vi "MHL_load file.vi"(0 "Data Cluster in":T1, 5 "error in (no error)":errorcluster) -> (14 "Data Cluster out":T1, 15 "Size (bytes)":i64=37399506 format="%.0p", 19 "error out":errorcluster)   [LabVIEW 2019, in "Main UI.lvlib"]
uses:
  Main UI.lvlib
  Module Data--cluster.ctl
  Neo-Laura-LVOOP/Class Library/XYgraph_class/XYgraph.lvclass
  FileReader/FPref_clustered--cluster references.ctl
  Main UI Shared/Boolean--FP cluster.ctl
  FileReader/FPref_cntrls--cluster references.ctl
  Main UI Shared/Indicators--FP cluster.ctl
  FileReader/FileReader.lvlib
  Analysis/Analysis.lvlib
  Main UI Shared/MAIN UI Shared.lvlib
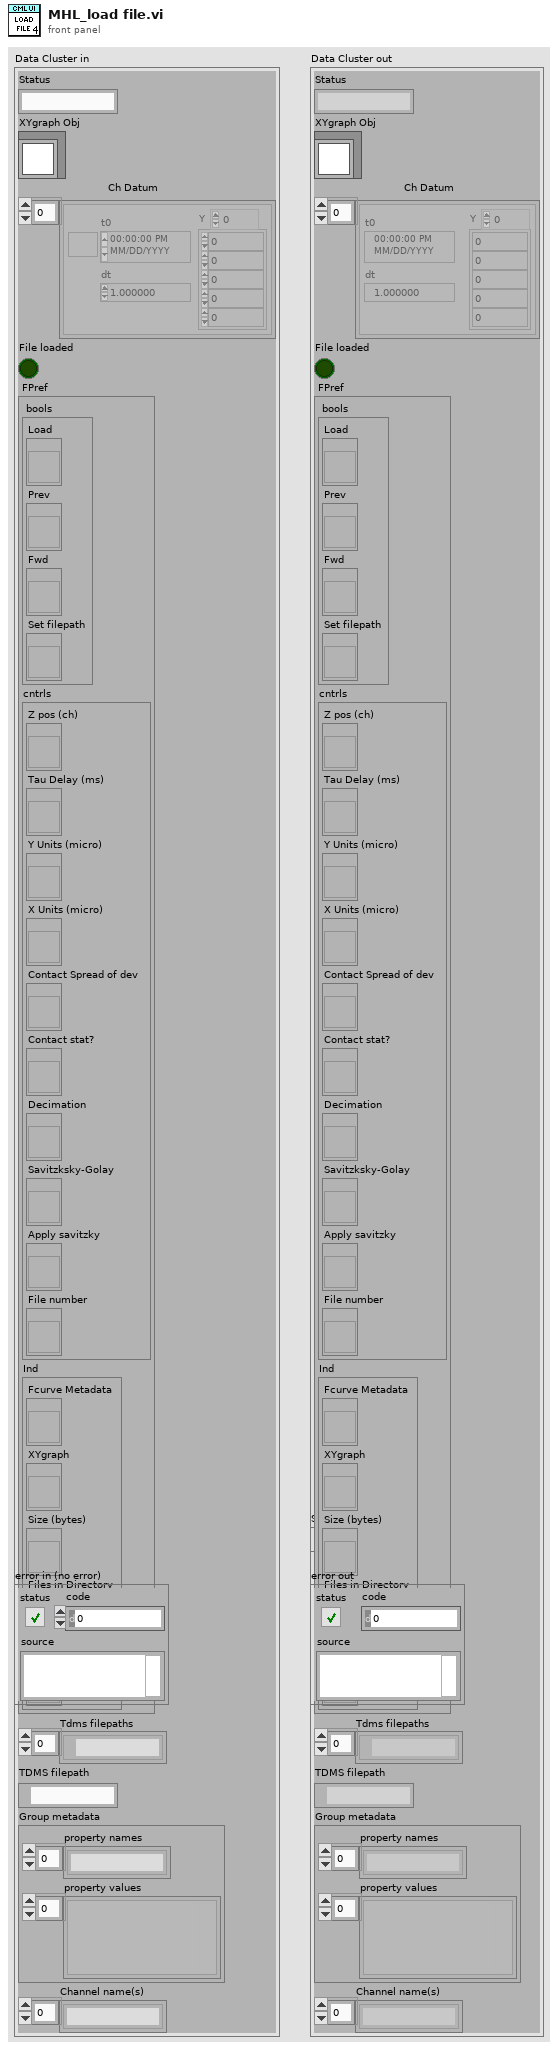
[diagram p1: front panel]
types:
  T1 = typedef "Main UI.lvlib/Module Data--cluster.ctl" = cluster{"Status":string, "XYgraph Obj":refnum<class "XYgraph.lvclass">, "Ch Datum":waveform(dbl)[], "File loaded":bool, "FPref":T2, "Tdms filepaths":path[], "TDMS filepath":path, "Group metadata":cluster{"property names":string[], "property values":variant[]}, "Channel name(s)":string[]}
  T2 = typedef "FPref_clustered--cluster references.ctl" = cluster{" bools":T3, "cntrls":T4, "Ind":T5}
  T3 = typedef "MAIN UI Shared.lvlib/Boolean--FP cluster.ctl" = cluster{"Load":refnum<vi>, "Prev":refnum<vi>, "Fwd":refnum<vi>, "Set filepath":refnum<vi>}
  T4 = typedef "FPref_cntrls--cluster references.ctl" = cluster{"Z pos (ch)":refnum<vi>, "Tau Delay (ms)":refnum<vi>, "Y Units (micro)":refnum<vi>, "X Units (micro)":refnum<vi>, "Contact Spread of dev":refnum<vi>, "Contact stat?":refnum<vi>, "Decimation":refnum<vi>, "Savitzksky-Golay":refnum<vi>, "Apply savitzky ":refnum<vi>, "File number":refnum<vi>}
  T5 = typedef "Indicators--FP cluster.ctl" = cluster{"Fcurve Metadata":refnum<vi>, "XYgraph":refnum<vi>, "Size (bytes)":refnum<vi>, "Files in Directory":refnum<vi>, "Filepath":refnum<vi>}
  T6 = typedef "MAIN UI Shared.lvlib/Apply_Savitsky--cluster.ctl" = cluster{"Def":bool, "Zpos":bool}
  T7 = typedef "FileReader.lvlib/Open TDMS file (Reply Payload)--cluster.ctl" = cluster{"Group metadata":T8, "Channel name(s)":string[], "Channel datum out":waveform(dbl)[], "size (in bytes)":i64, "error":errorcluster}
  T8 = typedef "TDMS_DataHandler.lvclass/Fcurve Meta data.ctl" = cluster{"property names":string[], "property values":variant[]}
  T9 = typedef "XYgraph.lvclass/Units --enum.ctl" = string
  T10 = typedef "Fcurve.lvclass/Metadata.ctl" = cluster{"dt (us)":dbl, "Dec Factor":dbl, "Z piezo Sensitivity (nm/V)":dbl, "K (N/m)":dbl, "Sp (V)":dbl, "Contact (ms)":dbl, "Zpos contact":dbl, "Vel_app (nm/s)":dbl, "Vel_ret (nm/s)":dbl, "deltaV (nm)":dbl, "Def_V0 (v)":dbl, "Piezo gain":dbl, "invOLS (nm/V)":dbl}
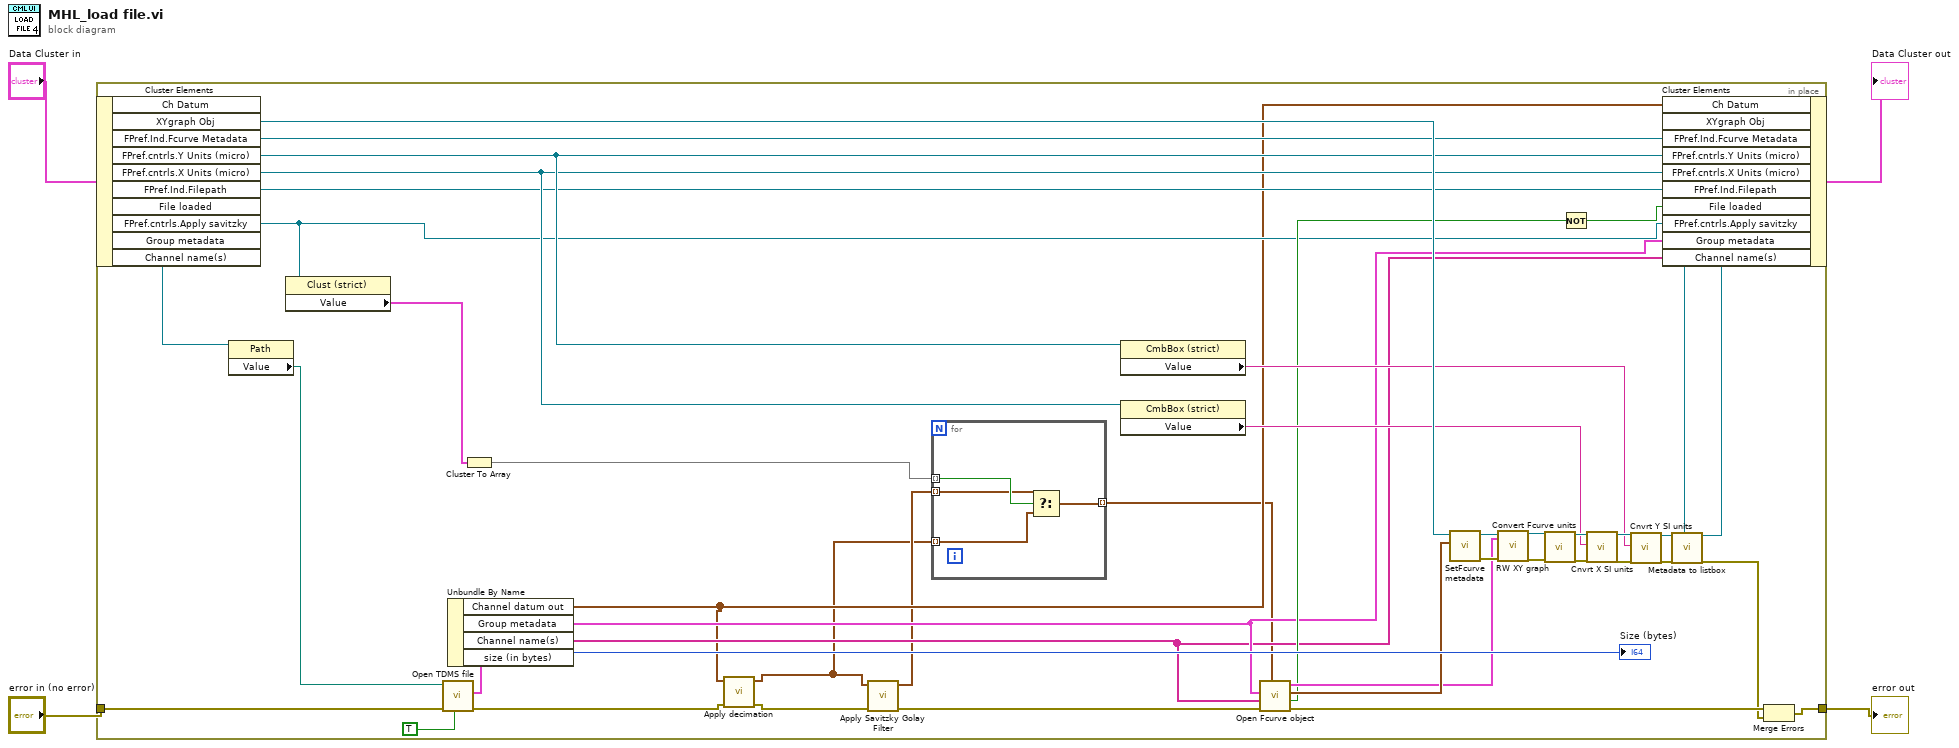
[diagram p0: block diagram]
diagram:
  n1 = in-place {
    in-place-border: "error in (no error)" -> [w46]
    in-place-border: [w39] -> w2
    n2 = in-place-cluster #1("Data Cluster in") -> ("XYgraph Obj"=w43:refnum<class "XYgraph.lvclass">, "FPref.Ind.Fcurve Metadata"=w26:refnum<vi>, "FPref.cntrls.Y Units (micro)"=w25:refnum<vi>, "FPref.cntrls.X Units (micro)"=w24:refnum<vi>, "FPref.Ind.Filepath"=w21:refnum<vi>, "FPref.cntrls.Apply savitzky"=w16:refnum<vi>)  [unwired: 4 out]
    n3 = property class="Path"(reference=w21) -> ("Value"=w20:path)  [unwired: 1 in, 2 out]
    n4 = property class="Clust (strict)"(reference=w16) -> ("Value"=w9:T6)  [unwired: 1 in, 2 out]
    n5 = call "Open TDMS file.vi"("wait for reply (T)"=TRUE, "error in"=w46, "TDMS filepath"=w20) -> ("error out"=w13:errorcluster, "Reply Payload"=w45:T7)  [unwired: 6 in, 1 out]
    n6 = Unbundle By Name(w45) -> ("Channel datum out"=w12:waveform(dbl)[], "Group metadata"=w15:T8, "Channel name(s)"=w14:string[], "size (in bytes)"=→"Size (bytes)":i64)
    n7 = Cluster To Array(cluster=w9) -> (array=w8:bool[])
    n8 = call "Apply decimation.vi"("error in"=w13, "Ch Datum"=w12) -> ("error out"=w11:errorcluster, "Wfms (wfms.array)"=w6:waveform(dbl)[])  [unwired: 7 in, 1 out]
    n9 = call "Apply Savitzky Golay Filter.vi"("error in"=w11, "Ch Datum"=w6) -> ("error out"=w10:errorcluster, "Filtered Ch Data"=w7:waveform(dbl)[])  [unwired: 7 in, 1 out]
    n10 = for {
      tunnel: w8 -> [w50] mode=indexing
      tunnel: w7 -> [w49] mode=indexing
      tunnel: w6 -> [w48] mode=indexing
      tunnel: [w47] -> w5 mode=indexing
      n11 = Select(t=w49, s=w50, f=w48) -> (s? t:f=w47:waveform(dbl))
    }
    n12 = property class="CmbBox (strict)"(reference=w25) -> ("Value"=w22:T9)  [unwired: 1 in, 2 out]
    n13 = property class="CmbBox (strict)"(reference=w24) -> ("Value"=w23:T9)  [unwired: 1 in, 2 out]
    n14 = call "Open Fcurve object.vi"("Channel datum out"=w5, "error in"=w10, "Channel name(s)"=w14, "Group metadata"=w15) -> ("error out"=w40:errorcluster, "timed out?"=w18:bool, "Metadata out"=w42:T10, "Fcurve out"=w37:cluster{"X":dbl[], "Y":dbl[]}[])  [unwired: 4 in]
    n15 = call-dynamic "SetFcurve metadata.vi"("Fcurve metadata"=w42, "reference in"=w43) -> ("error out"=w38:errorcluster, "reference out"=w41:refnum<class "XYgraph.lvclass">)  [unwired: 8 in]
    n16 = call-dynamic "RW XY graph.vi"("reference in"=w41, "XY in"=w37, "error in (no error)"=w38) -> ("reference out"=w36:refnum<class "XYgraph.lvclass">, "error out"=w32:errorcluster)  [unwired: 14 in, 1 out]
    n17 = call-dynamic "Convert Fcurve units.vi"("reference in"=w36, "error in (no error)"=w32) -> ("reference out"=w33:refnum<class "XYgraph.lvclass">, "error out"=w31:errorcluster)  [unwired: 16 in]
    n18 = Not(x=w18) -> (.not. x?=w17:bool)
    n19 = call-dynamic "Cnvrt X SI units.vi"("reference in"=w33, "X Units (micro)"=w23, "error in (no error)"=w31) -> ("reference out"=w35:refnum<class "XYgraph.lvclass">, "error out"=w34:errorcluster)  [unwired: 15 in]
    n20 = call-dynamic "Cnvrt Y SI units.vi"("reference in"=w35, "Units (micro)"=w22, "error in (no error)"=w34) -> ("reference out"=w30:refnum<class "XYgraph.lvclass">, "error out"=w28:errorcluster)  [unwired: 15 in]
    n21 = call-dynamic "Metadata to listbox.vi"("reference in"=w30, "error in (no error)"=w28, "Fcurve Metadata ref"=w26) -> ("reference out"=w29:refnum<class "XYgraph.lvclass">, "error out"=w27:errorcluster)  [unwired: 14 in, 1 out]
    n22 = in-place-cluster #1("Ch Datum"=w12, "XYgraph Obj"=w29, "FPref.Ind.Fcurve Metadata"=w26, "FPref.cntrls.Y Units (micro)"=w25, "FPref.cntrls.X Units (micro)"=w24, "FPref.Ind.Filepath"=w21, "File loaded"=w17, "FPref.cntrls.Apply savitzky"=w16, "Group metadata"=w15, "Channel name(s)"=w14) -> (→"Data Cluster out":T1)
    n23 = Merge Errors(w40, w27) -> (w39:errorcluster)
  }
  "error out" <- w2
